vi "LWXPS_Close.vi"(3 "error in (no error)":errorcluster caption="error in", 5 "XPS Reference":refnum<k24>) -> (0 "Error out":errorcluster caption="error out", 1 "Error code":i32)   [LabVIEW 2020]
uses:
  C:/GEECS/Developers Version/source/Device Drivers/NewportXPS/XPS-RLD/XPS-UNIFIED/LabVIEW VIs/Sample Project/Dll/Newport.XPS.CommandInterface.dll
  Dll/Newport.XPS.CommandInterface.dll
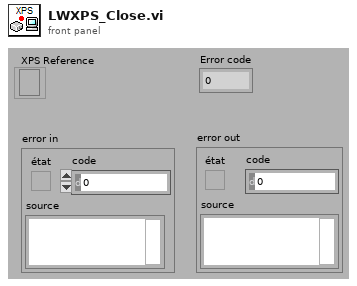
[diagram p1: front panel]
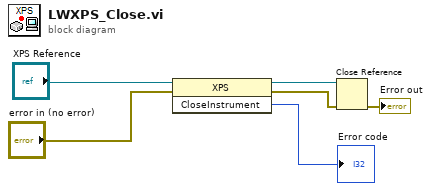
[diagram p0: block diagram]
diagram:
  n1 = invoke class="XPS" method="CloseInstrument"(reference="XPS Reference", error in="error in (no error)") -> (reference out=w6:refnum<k24>, error out=w5:errorcluster, "CloseInstrument"=→"Error code":i32)  [unwired: 1 in]
  n2 = Close Reference(reference=w6, error in (no error)=w5) -> (error out=→"Error out":errorcluster)
